vi "observacao_queued.vi"() -> ()   [LabVIEW 2012, in "Shared_160.lvlib"] (continued)
                n273 = local write "sendCommandShutter"(FALSE ("writeShutterLog")) -> ()
                n274 = call "Monta Comando.vi"("Comando"="PARAR", "Dispositivo"="TRAPEIRA" ("Comando"), "Controlador"=w182) -> ()  [unwired: 4 in, 3 out]
              }
            }
            n275 = local read "MOVING"() -> (w97:bool)
            n276 = global write "Global_Telescopio.vi" "Sideral Time"(w114) -> ()
            n277 = Or(x=w96, y=w97) -> (x .or. y?=w95:bool)
            n278 = shared-variable "My Computer\\Shared_160.lvlib\\Beep"(w95) -> ()  [unwired: 1 in, 1 out]
          }
          frame #1 {
            w268 = u16 9 items=["Alarme", "Atencao", "Erro", "Ocupado", "Protecao", "Embreagem", "Tracking", "Var. Track", "Rápido", "Ligeiro", "Médio", "Lento", "Em movimento", ""] ("NomeStatus")
            w269 = u16 9 items=["Alarme", "Atencao", "Erro", "Ocupado", "Protecao", "Embreagem", "Tracking", "Var. Track", "Rápido", "Ligeiro", "Médio", "Lento", "Em movimento", ""] ("NomeStatus")
            w272 = u16 8 items=["Alarme", "Atencao", "Erro", "Ocupado", "Protecao", "Embreagem", "Tracking", "Var. Track", "Rápido", "Ligeiro", "Médio", "Lento", "Em movimento", ""] ("NomeStatus")
            w273 = u16 8 items=["Alarme", "Atencao", "Erro", "Ocupado", "Protecao", "Embreagem", "Tracking", "Var. Track", "Rápido", "Ligeiro", "Médio", "Lento", "Em movimento", ""] ("NomeStatus")
            w279 = 6.283185307179586
            # "Desabilita botões \"Precess\" e \"Clear\"\ndurante o apontamento"
            # "MUDANÇA:\nBit EMBREAGEM trocado pelos bits RAPIDO e LIGEIRO para detectar a retirada do objeto da posição centrada."
            # "MUDANÇA FUTURA:\nTrocar globais de calagem por valores \"latch\" dessas globais. Finalidade: manter display de coordenadas consistentes mesmo quando o usuário zerar as calagens, especialmente a local, para o próximo apontamento."
            # "ATUALIZA INDICADORES DO PAINEL"
            n279 = local read "ChkCalGlobal"() -> (w284:bool)
            n280 = global read "Global_Telescopio.vi" "PosDEC"() -> (w287:dbl)
            n281 = global read "Global_Telescopio.vi" "Sideral Time"() -> (w289:dbl)
            n282 = global read "Global_Telescopio.vi" "ObjCentrado"() -> (w260:bool)
            "ObjCentrado" <- w260
            n283 = global read "Global_Telescopio.vi" "PosAH"() -> (w288:dbl)
            n284 = call "Calcula epoch.vi"() -> ("epoch"=→"Epoch":dbl)  [unwired: 2 in]
            n285 = call "Bit Status AH.vi"("NomeStatus"=w273) -> ("StatBit"=w271:bool)
            n286 = call "Bit Status AH.vi"("NomeStatus"=w268) -> ("StatBit"=w267:bool)
            n287 = call "Bit Status DEC.vi"("NomeStatus"=w272) -> ("StatBit"=w265:bool)
            n288 = call "Bit Status DEC.vi"("NomeStatus"=w269) -> ("StatBit"=w266:bool)
            n289 = Compound Arithmetic op=OR(w271, w267, w265, w266) -> (w270:bool)
            n290 = case shown="True" w270 {
              frame False {
              }
              frame True {
                n291 = global write "Global_Telescopio.vi" "ObjCentrado"(FALSE) -> ()
              }
            }
            n292 = Tick Count (ms)() -> (millisecond timer value=w256:u32)
            n293 = local read "LedPointing"() -> (w255:bool)
            n294 = case shown="True" w260 {
              tunnel: [w366 w383] -> w281
              tunnel: [w365 w382] -> w277
              tunnel: [w368 w386] -> w261
              tunnel: [w367 w384] -> w274
              tunnel: w289 -> [w366 w383]
              tunnel: w288 -> [w371 _]
              tunnel: w287 -> [w370 _]
              tunnel: w284 -> [w369 _]
              tunnel: [w364 w380] -> _
              tunnel: w256 -> [w364 w380]
              frame False {
                n295 = case shown="False" w369 {
                  tunnel: w370 -> [w373 w379]
                  tunnel: [w373 w378] -> w368
                  tunnel: w371 -> [w372 w377]
                  tunnel: [w372 w374] -> w367
                  frame False {
                  }
                  frame True {
                    n296 = global read "Global_Telescopio.vi" "Calagem AH"() -> (w375:dbl)
                    n297 = global read "Global_Telescopio.vi" "Calagem DEC"() -> (w376:dbl)
                    n298 = Subtract(x=w377, y=w375) -> (x-y=w374:dbl)
                    n299 = Subtract(x=w379, y=w376) -> (x-y=w378:dbl)
                  }
                }
                n300 = Subtract(x=w366, y=w367) -> (x-y=w365:dbl)
              }
              frame True {
                # "PROCESSO PRECESSÃO"
                n301 = local read "Temp amb"() -> (w389:string)
                n302 = local read "hum local"() -> (w387:string)
                n303 = local read "MeanDEC"() -> (w390:string)
                n304 = local read "pressão atm"() -> (w388:string)
                n305 = local read "PM_RA"() -> (w385:string)
                n306 = local read "MeanRA"() -> (w391:string)
                n307 = local read "PM_DEC"() -> (w381:string)
                n308 = call "PrecessFortran.vi"("Asc reta"=w391, "Var RA"=w385, "Declinação"=w390, "Temperatura (Kelvin)"=w389, "Pressao atmosferica (mB)"=w388, "Humidade relativa (0 a 1)"=w387, "Var DEC"=w381) -> ("Observed RA (radians)"=w382:dbl, "Observed Dec (radians)"=w386:dbl)  [unwired: 2 in, 5 out]
                n309 = Subtract(x=w383, y=w382) -> (x-y=w384:dbl)
              }
            }
            "AtualDEC" <- w261
            n310 = case shown="True" w260 {
              tunnel: w261 -> [_ w320]
              tunnel: [w317 w319] -> w286
              tunnel: [w317 w318] -> w285
              frame False {
                w317 = 0.0
              }
              frame True {
                n311 = stacked-sequence {
                  seq-local: [w321 _ _] -> [_ _ w359]
                  tunnel: w320 -> [_ w328 _]
                  tunnel: [_ w327 _] -> w319
                  tunnel: [_ w326 _] -> w318
                  frame #0 {
                    n312 = Tick Count (ms)() -> (millisecond timer value=w321:u32)
                  }
                  frame #1 {
                    w329 = u16 3 items=["Alarme", "Atencao", "Erro", "Ocupado", "Protecao", "Embreagem", "Tracking", "Var. Track", "Rápido", "Ligeiro", "Médio", "Lento", "Em movimento", ""] ("NomeStatus")
                    w330 = u16 3 items=["Alarme", "Atencao", "Erro", "Ocupado", "Protecao", "Embreagem", "Tracking", "Var. Track", "Rápido", "Ligeiro", "Médio", "Lento", "Em movimento", ""] ("NomeStatus")
                    # "PROCESSO LEITURA POS_MOTOR"
                    n313 = local read "MOV_IDX_AH"() -> (w324:bool)
                    n314 = local read "MOV_IDX_DEC"() -> (w322:bool)
                    n315 = call "Bit Status AH.vi"("NomeStatus"=w330) -> ("StatBit"=w325:bool)
                    n316 = call "Bit Status DEC.vi"("NomeStatus"=w329) -> ("StatBit"=w323:bool)
                    n317 = case shown="False" w325 {
                      tunnel: w328 -> [w344 _]
                      tunnel: [w343 w358] -> w327
                      tunnel: w324 -> [w342 _]
                      frame False {
                        n318 = case shown="False" w342 {
                          tunnel: w344 -> [w352 _]
                          tunnel: [w348 w357] -> w343
                          frame False {
                            w355 = u16 1 items=["ZERO", "AH", "DEC", "TUBO", "CUP"] ("Controlador")
                            # "RA"
                            # "AH"
                            n319 = call "Get Posic Motor Indexer.vi"("Controlador"=w355) -> ("PosMotor"=w346:dbl)
                            n320 = global read "Global_Telescopio.vi" "AcumPrecRA"() -> (w349:dbl)
                            n321 = Negate(x=w346) -> (-x=w347:dbl)
                            n322 = Subtract(x=w347, y=w349) -> (x-y=w356:dbl)
                            n323 = global read "Global_Telescopio.vi" "AcumAG RA"() -> (w350:dbl)
                            n324 = Cosine(x=w352) -> (cos(x)=w351:dbl)
                            n325 = Absolute Value(x=w351) -> (abs(x)=w345:dbl)
                            n326 = Subtract(x=w356, y=w350) -> (x-y=w354:dbl)
                            n327 = Multiply(x=w345, y=w354) -> (x*y=w353:dbl)
                            n328 = call "Rad to Arcsec.vi"("Radiano"=w353) -> ("Arcsec"=w348:dbl)
                          }
                          frame True {
                            n329 = local read "Offset RA"() -> (w357:dbl)
                          }
                        }
                      }
                      frame True {
                        n330 = local read "Offset RA"() -> (w358:dbl)
                      }
                    }
                    n331 = case shown="False" w323 {
                      tunnel: [w332 w341] -> w326
                      tunnel: w322 -> [w331 _]
                      frame False {
                        n332 = case shown="False" w331 {
                          tunnel: [w333 w340] -> w332
                          frame False {
                            w336 = u16 2 items=["ZERO", "AH", "DEC", "TUBO", "CUP"] ("Controlador")
                            n333 = call "Get Posic Motor Indexer.vi"("Controlador"=w336) -> ("PosMotor"=w338:dbl)
                            n334 = global read "Global_Telescopio.vi" "AcumPrecDEC"() -> (w334:dbl)
                            n335 = Subtract(x=w338, y=w334) -> (x-y=w339:dbl)
                            n336 = global read "Global_Telescopio.vi" "AcumAG DEC"() -> (w335:dbl)
                            n337 = Subtract(x=w339, y=w335) -> (x-y=w337:dbl)
                            n338 = call "Rad to Arcsec.vi"("Radiano"=w337) -> ("Arcsec"=w333:dbl)
                          }
                          frame True {
                            n339 = local read "Offset DEC"() -> (w340:dbl)
                          }
                        }
                      }
                      frame True {
                        n340 = local read "Offset DEC"() -> (w341:dbl)
                      }
                    }
                  }
                  frame #2 {
                    n341 = flat-sequence {
                      tunnel: w359 -> [w360]
                      frame #0 {
                        n342 = Tick Count (ms)() -> (millisecond timer value=w361:u32)
                        n343 = Subtract(x=w361, y=w361) -> (x-y=→"dtAUX2":u32)
                        n344 = Subtract(x=w361, y=w360) -> (x-y=→"dtAUX3":u32)
                      }
                    }
                  }
                }
              }
            }
            "Offset RA" <- w286
            "Offset DEC" <- w285
            n345 = case shown="False" w255 {
              frame False {
                w295 = 0
                n346 = property on="BtPointPrecess" class="Bool"("DisabledEnum"=w295) -> ()  [unwired: 2 in, 2 out]
                n347 = property on="BtPointObjClear" class="Bool"("DisabledEnum"=w295) -> ()  [unwired: 2 in, 2 out]
              }
              frame True {
                w296 = 2
                n348 = property on="BtPointPrecess" class="Bool"("DisabledEnum"=w296) -> ()  [unwired: 2 in, 2 out]
                n349 = property on="BtPointObjClear" class="Bool"("DisabledEnum"=w296) -> ()  [unwired: 2 in, 2 out]
              }
            }
            n350 = call "Normliza_AH.vi"("PosAH"=w274) -> ("Numeric"=w259:dbl)
            n351 = Add(x=w279, y=w277) -> (x+y=w278:dbl)
            n352 = Add(x=w279, y=w281) -> (x+y=w282:dbl)
            n353 = Less Than 0?(x=w281) -> (x < 0?=w283:bool)
            n354 = Less Than 0?(x=w277) -> (x < 0?=w280:bool)
            n355 = Select(t=w282, s=w283, f=w281) -> (s? t:f=w262:dbl)
            n356 = Select(t=w278, s=w280, f=w277) -> (s? t:f=w263:dbl)
            n357 = case shown="True" w260 {
              tunnel: ["" w304] -> w264
              tunnel: w263 -> [_ w301]
              tunnel: w262 -> [_ w302]
              tunnel: w261 -> [_ w303]
              frame False {
              }
              frame True {
                n358 = disable-structure shown="Disabled" {
                  disable-tunnel: w303 -> [w315 _]
                  disable-tunnel: w302 -> [w314 _]
                  disable-tunnel: w301 -> [w313 _]
                  disable-tunnel: [w312 _] -> _
                  frame Disabled {
                    n359 = call "Hora_Limite.vi"("Asc Reta RA rad"=w313, "Sideral Time rad"=w314, "Declinação rad"=w315) -> ("TO Tempo de Observação Horas"=w312:dbl)  [unwired: 2 in]
                  }
                  frame Enabled {
                  }
                }
                n360 = call "Novo_tempo_obs.vi"() -> ("TO rad"=w299:dbl)  [unwired: 10 in, 1 out]
                n361 = Greater Than 0?(x=w299) -> (x > 0?=w298:bool)
                n362 = case shown="True" w298 {
                  tunnel: [w306 w309] -> w300
                  tunnel: w299 -> [w306 w308]
                  frame False {
                  }
                  frame True {
                    n363 = Random Number (0-1)() -> (number: 0 to 1=w310:dbl)
                    n364 = Multiply(x=w310, y=7.27e-05) -> (x*y=w307:dbl)
                    n365 = Add(x=w308, y=w307) -> (x+y=w309:dbl)
                  }
                }
                n366 = call "rad_hms.vi"("TRUE=HORA\nFALSE=GRAU"=TRUE ("TRUE=HORA\nFALSE=GRAU"), "Radiano"=w300) -> ("Hora/Graus Texto Decimal"=w304:string)  [unwired: 3 in]
              }
            }
            "Time to Limit" <- w264
            n367 = call "rad_hms.vi"("TRUE=HORA\nFALSE=GRAU"=TRUE ("TRUE=HORA\nFALSE=GRAU"), "Radiano"=w262) -> ("Hora/Graus Texto Decimal"=w276:string)  [unwired: 3 in]
            "Sideral time" <- w276
            n368 = call "rad_hms.vi"("TRUE=HORA\nFALSE=GRAU"=TRUE, "Radiano"=w263) -> ("Hora/Graus Texto Decimal"=w275:string)  [unwired: 3 in]
            "Right Ascention" <- w275
            n369 = call "rad_hms.vi"("TRUE=HORA\nFALSE=GRAU"=TRUE, "Radiano"=w259) -> ("Hora/Graus Texto Decimal"=w258:string)  [unwired: 3 in]
            "Hour Angle" <- w258
            "Hour Angle 2" <- w258
            n370 = call "rad_hms.vi"("TRUE=HORA\nFALSE=GRAU"=FALSE, "Radiano"=w261) -> ("Hora/Graus Texto Decimal"=w257:string)  [unwired: 3 in]
            "Declination" <- w257
            "DEC" <- w257
            n371 = global write "Global_Telescopio.vi" "Right Ascention"(w275) -> ()
            n372 = global write "Global_Telescopio.vi" "Hour Angle"(w258) -> ()
            n373 = global write "Global_Telescopio.vi" "Sideral time"(w276) -> ()
            n374 = global write "Global_Telescopio.vi" "Declination"(w257) -> ()
            n375 = global write "Global_Telescopio.vi" "AH_now"(w259) -> ()
            n376 = global write "Global_Telescopio.vi" "delta_now"(w261) -> ()
          }
          frame #2 {
            w416 = -0.39330025  # LatOPD rad
            # "ALTERAÇÃO FEITA EM 12/12/2012\nFEITA PARA RESOLVER EXCESSÍVOS\nMOVIMENTOS DO ACOMP.SID. DA\nCÚPULA (DANIEL). A condição de statCUP=0 foi inserida em 08/5/2013-> Só corrige a cúpula se esta estiver parada!"
            # "Horas"
            # "MUDANÇA FUTURA:\nPassar LatOPD para Global"
            # "az"
            # "z"
            # "Cálculo do Azimute da Cúpula e Hab Acompanham. Cúpula"
            # "Lógica de Segurança"
            # "ANGULO ZENITAL"
            n377 = global read "Global_Telescopio.vi" "OffsetCupula"() -> (w425:dbl)
            n378 = global read "Global_Telescopio.vi" "AH_now"() -> (w407:dbl)
            n379 = global read "Global_Telescopio.vi" "delta_now"() -> (w415:dbl)
            n380 = global read "Global_Telescopio.vi" "ErroMaxCup"() -> (w394:i16)
            n381 = global read "Global_Telescopio.vi" "Limite EAST"() -> (w408:dbl)
            n382 = global read "Global_Telescopio.vi" "Limite WEST"() -> (w409:dbl)
            n383 = global read "Global_Telescopio.vi" "PosCUP"() -> (w395:i16)
            "PosCUP" <- w395
            n384 = local read "Tick Cupula"() -> (w399:u32)
            n385 = call "Calculo_do_Azimute_da_Cupula_2.vi"("AH"=w407, "DEC"=w415, "OffsetTCSPD"=w425) -> ("PosCup"=w392:u16)  [unwired: 3 in, 1 out]
            "Azimute cup" <- w392
            n386 = Tick Count (ms)() -> (millisecond timer value=w400:u32)
            n387 = Multiply(x=w407, y=3.8197) -> (x*y=w410:dbl)
            n388 = call "Altura_e_Azimute.vi"("LAT rad"=w416, "DEC rad"=w415, "AH rad"=w407) -> ("AZIMUTE graus"=w413:dbl, "ANG. ZENITAL graus"=w414:dbl, "AZIMUTE rad"=w417:dbl, "ANG. ZENITAL rad"=w418:dbl)  [unwired: 2 out]
            "Azimuth" <- w413
            "Zenital angle" <- w414
            n389 = Greater Or Equal?(x=w400, y=w399) -> (x >= y?=w398:bool)
            n390 = Greater?(x=w410, y=w408) -> (0:w406:bool)
            n391 = Less?(x=w410, y=w409) -> (x < y?=w405:bool)
            n392 = call "Verifica_Correcao_CUP.vi"("Erro max"=w394, "Pos Atual"=w395, "Azimute"=w392) -> ("Corrigir?"=w393:bool)  [unwired: 2 in]
            n393 = Not And(1:w405, 2:w406) -> (0:w402:bool)
            n394 = local read "statCUP"() -> (w397:i32)
            n395 = call "Calcula_Proteção.vi"("Zenital angle rad"=w418, "Azimute rad"=w417) -> ("Z_SEGURANÇA_GRAUS"=w427:dbl, "Prot Segur"=w429:bool, "Z_LIBERA_GRAUS"=w426:dbl, "Z_MAX_GRAUS"=w428:dbl, "Prot Zmax"=w403:bool)
            n396 = Equal To 0?(x=w397) -> (x = 0?=w396:bool)
            n397 = global write "Global_Telescopio.vi" "Z_SEGURANÇA_GRAUS"(w427) -> ()
            n398 = global write "Global_Telescopio.vi" "Zenital angle GRAUS"(w414) -> ()
            n399 = global write "Global_Telescopio.vi" "Azimute GRAUS"(w413) -> ()
            n400 = global write "Global_Telescopio.vi" "Z_MAX_GRAUS"(w428) -> ()
            n401 = global write "Global_Telescopio.vi" "Z_LIBERA_GRAUS"(w426) -> ()
            n402 = Compound Arithmetic op=AND(w393, "DOME", w398, w396) -> (w424:bool)
            n403 = case shown="True" w424 {
              tunnel: w392 -> [_ w438]
              tunnel: FALSE -> [_ w436]
              frame False {
              }
              frame True {
                # "TEMPO CÚPULA"
                # "2m Tempo para novo movimento"
                n404 = local write "Dome on Target"(w436) -> ()
                n405 = Tick Count (ms)() -> (millisecond timer value=w435:u32)
                n406 = To Word Integer(number=w438) -> (16bit integer=w432:i16)
                n407 = local write "statCUP"(1 ("statCUP")) -> ()
                n408 = Add(x=w435, y=u32 120000) -> (x+y=→"Tick Cupula":u32)
                n409 = global write "Global_Telescopio.vi" "TargetCUP"(w432) -> ()
              }
            }
            n410 = Or(x=w402, y=w403) -> (x .or. y?=w404:bool)
            n411 = global read "Global_Telescopio.vi" "LIMITE"() -> (w423:bool)
            n412 = Or(x=w423, y=w404) -> (x .or. y?=w422:bool)
            "Proteção" <- w422
            n413 = call "Borda_Subida_Segurança.vi"("Entrada"=w429) -> ("Boolean"=w430:bool)
            n414 = call "Borda_Subida_Z_max.vi"("Entrada"=w422) -> ("Boolean"=w431:bool)
            n415 = Select(t=u8 2 ("Disabled"), s=w422, f=u8 0 ("Disabled")) -> (s? t:f=w419:u8)
            n416 = property on="MOUNT" class="Bool (strict)"("Disabled"=w419) -> ()  [unwired: 2 in, 2 out]
            n417 = case shown="True" w430 {
              frame False {
              }
              frame True {
                w441 = u16 2 items=["ZERO", "AH", "DEC", "TUBO", "CUP"] ("Controlador")
                w440 = "FREAR" ("Comando")
                w442 = u16 1 items=["ZERO", "AH", "DEC", "TUBO", "CUP"] ("Controlador")
                w439 = "EIXO" ("Dispositivo")
                n418 = call "Monta Comando.vi"("Comando"=w440, "Dispositivo"=w439, "Controlador"=w442) -> ()  [unwired: 4 in, 3 out]
                n419 = call "Monta Comando.vi"("Comando"=w440, "Dispositivo"=w439, "Controlador"=w441) -> ()  [unwired: 4 in, 3 out]
              }
            }
            n420 = case shown="True" w431 {
              frame False {
              }
              frame True {
                w445 = FALSE
                w443 = "Telescópio parado por inclinação excessiva!" ("SYSTEM MESSAGES")
                n421 = local write "LED MOUNT"(w445) -> ()
                n422 = local write "MOUNT"(w445) -> ()
                n423 = global write "Global_Telescopio.vi" "ObjCentrado"(FALSE) -> ()
                n424 = global write "Global_Telescopio.vi" "STOP ALL"(TRUE ("STOP ALL")) -> ()
                n425 = call "Monta_Mensagem.vi"("Mensagem"=w443) -> ()  [unwired: 2 in]
                n426 = call "Salva_systems_messages.vi"("Mensagem"=w443) -> ()  [unwired: 5 in]
              }
            }
            "Led Chave Dome" <- "DOME"
          }
          frame #3 {
            w452 = u32 500 ("millisecond multiple")
            w466 = u16 3 items=["Alarme", "Atencao", "Erro", "Ocupado", "TBD", "LCB", "Trapeira", "Paravento", "DomoRap", "DomoCW", "DomoCCW", "TBD", "Em movimento", "TBD"] ("NomeStatus")
            w480 = u16 3 items=["Alarme", "Atencao", "Erro", "Ocupado", "Protecao", "Embreagem", "Tracking", "Var. Track", "Rápido", "Ligeiro", "Médio", "Lento", "Em movimento", ""] ("NomeStatus")
            w481 = u16 3 items=["Alarme", "Atencao", "Erro", "Ocupado", "Protecao", "Embreagem", "Tracking", "Var. Track", "Rápido", "Ligeiro", "Médio", "Lento", "Em movimento", ""] ("NomeStatus")
            # "04-07-2022\nValor de Erro PROTEC\nalterado de 5 para 10"
            # "MUDANÇA: \nIncluído CASE"
            # "Esse metrônomo determina\no ciclo de 0,5 segundo dos\ncálculos rápidos e totais!"
            # "PROCESSO APONTAMENTO"
            # "MÁQUINA DE ESTADO DO APONTAMENTO"
            # "Seta nome para GO/STOP"
            n427 = global read "Global_Telescopio.vi" "LimiarRapMed"() -> (w482:dbl)
            n428 = global write "Global_Telescopio.vi" "Estado DEC"("statDEC") -> ()
            n429 = global read "Global_Telescopio.vi" "Sideral Time"() -> (w460:dbl)
            n430 = global read "Global_Telescopio.vi" "PosAH"() -> (w485:dbl)
            n431 = global read "Global_Telescopio.vi" "ErroMaxEixo"() -> (w469:dbl)
            n432 = global read "Global_Telescopio.vi" "PosDEC"() -> (w483:dbl)
            n433 = global read "Global_Telescopio.vi" "TargetRA"() -> (w486:dbl)
            n434 = global read "Global_Telescopio.vi" "TargetDEC"() -> (w484:dbl)
            n435 = call "Bit Status DEC.vi"("NomeStatus"=w480) -> ("StatBit"=w468:bool)
            n436 = call "Bit Status AH.vi"("NomeStatus"=w481) -> ("StatBit"=w467:bool)
            n437 = case shown="4" "statDEC" {
              selector: "statDEC" -> [w615 _ _ _ _ _ _ _ _]
              tunnel: [w615 w622 w652 w674 w701 w725 0 ("t") w742 w747] -> w461
              tunnel: w484 -> [_ w621 _ w668 _ _ _ _ _]
              tunnel: w483 -> [_ w617 _ w671 _ _ _ _ _]
              tunnel: w469 -> [_ _ _ w672 _ _ _ _ _]
              tunnel: w482 -> [_ w623 _ _ _ _ _ _ _]
              tunnel: w468 -> [_ w620 _ w667 _ _ _ _ _]
              frame 0, Default {
                w613 = 0 ("CR DEC")
                # "Sem apontamento"
                n438 = call "TickTimeout.vi"() -> ("msTick"=→"TimeoutDEC":u32)  [unwired: 2 in, 2 out]
                n439 = local write "CR DEC"(w613) -> ()
                n440 = local write "C. DEC"(w613) -> ()
              }
              frame 1 {
                # "Envia\nComando"
                n441 = Subtract(x=w621, y=w617) -> (x-y=w619:dbl)
                n442 = Absolute Value(x=w619) -> (abs(x)=w624:dbl)
                n443 = Less?(x=w624, y=w623) -> (x < y?=w618:bool)
                n444 = case shown="False" w618 {
                  tunnel: [w628 3] -> w622
                  tunnel: w621 -> [w627 _]
                  tunnel: w619 -> [w626 _]
                  tunnel: w620 -> [w625 _]
                  frame False {
                    # "destino"
                    # "Fora do"
                    n445 = case shown="False" w625 {
                      tunnel: [w632 w640] -> w628
                      tunnel: w627 -> [w635 _]
                      tunnel: w626 -> [_ _]
                      frame False {
                        w639 = u16 2 items=["ZERO", "AH", "DEC", "TUBO", "CUP"] ("Controlador")
                        # "limpa flag"
                        # "CLP Pronto"
                        n446 = local write "Flag ativo DEC"(FALSE ("Flag ativo DEC")) -> ()
                        n447 = call "rad_hms.vi"("TRUE=HORA\nFALSE=GRAU"=FALSE, "Radiano"=w635) -> ("Hora/Graus Texto Decimal"=w636:string)  [unwired: 3 in]
                        n448 = call "Monta Comando.vi"("Set Point"=w636, "Comando"="MOVER_RAP", "Dispositivo"="EIXO" ("Comando"), "Controlador"=w639) -> ("Erro Comunicação"=w630:bool)  [unwired: 3 in, 2 out]
                        n449 = Select(t=6, s=w630, f=20) -> (s? t:f=w632:i32)
                      }
                      frame True {
                        # "CLP Ocupado"
                        n450 = local read "TimeoutDEC"() -> (w642:u32)
                        n451 = call "TickTimeout.vi"("msInicial"=w642, "msTimeout"=u32 4000) -> ("Timeout"=w641:bool)  [unwired: 2 out]
                        n452 = case shown="False" w641 {
                          tunnel: [1 5] -> w640
                          frame False {
                          }
                          frame True {
                            # "Tratar\nTimeout"
                          }
                        }
                      }
                    }
                  }
                  frame True {
                    # "Dist. pequena p/ mov. rápido"
                    # "Ligar mov. lento"
                    n453 = call "TickTimeout.vi"() -> ("msTick"=w646:u32)  [unwired: 2 in, 2 out]
                    n454 = local write "TimeoutDEC"(w646) -> ()
                  }
                }
                n455 = local write "dec="(FALSE ("dec=")) -> ()
              }
              frame 2 {
                w653 = u16 12 items=["Alarme", "Atencao", "Erro", "Ocupado", "Protecao", "Embreagem", "Tracking", "Var. Track", "Rápido", "Ligeiro", "Médio", "Lento", "Em movimento", ""] ("NomeStatus")
                # "Aguarda fim mov. Rap."
                n456 = call "Bit Status DEC.vi"("NomeStatus"=w653) -> ("StatBit"=w654:bool)
                n457 = case shown="True" w654 {
                  tunnel: [1 w663] -> w651
                  frame False {
                    # "Motor parado.\nTestar se chegou\nao destino"
                    n458 = call "TickTimeout.vi"() -> ("msTick"=w659:u32)  [unwired: 2 in, 2 out]
                    n459 = local write "TimeoutDEC"(w659) -> ()
                  }
                  frame True {
                    # "Ainda movendo...\nAGUARDAR"
                    n460 = local read "Erro PROTEC"() -> (w665:i32)
                    n461 = call "PROTECAO_DEC.vi"() -> ("CONT DEC"=w666:i32)  [unwired: 11 in]
                    "C. DEC" <- w666
                    n462 = Greater Or Equal?(x=w666, y=w665) -> (x >= y?=w661:bool)
                    n463 = Select(t=6, s=w661, f=2) -> (s? t:f=w663:i32)
                  }
                }
                n464 = global read "Global_Telescopio.vi" "Habilita supervisao"() -> (w649:bool)
                n465 = case shown="True" w649 {
                  tunnel: [FALSE w658] -> w648
                  frame False {
                  }
                  frame True {
                    n466 = local read "Erro Lim"() -> (w656:i32)
                    n467 = Greater Or Equal?(x="CR DEC", y=w656) -> (x >= y?=w658:bool)
                  }
                }
                n468 = Select(t=6, s=w648, f=w651) -> (s? t:f=w652:i32)
              }
              frame 3 {
                # "Mov.Lento"
                n469 = Subtract(x=w668, y=w671) -> (x-y=w669:dbl)
                n470 = Absolute Value(x=w669) -> (abs(x)=w673:dbl)
                n471 = Less Or Equal?(x=w673, y=w672) -> (x <= y?=w670:bool)
                n472 = case shown="False" w670 {
                  selector: w670 -> [_ w697]
                  tunnel: [w676 0] -> w674
                  tunnel: w669 -> [w675 _]
                  tunnel: w668 -> [_ w696]
                  tunnel: w667 -> [w677 _]
                  frame False {
                    n473 = case shown="False" w677 {
                      tunnel: [w681 w690] -> w676
                      tunnel: w675 -> [w684 _]
                      frame False {
                        w689 = u16 2 items=["ZERO", "AH", "DEC", "TUBO", "CUP"] ("Controlador")
                        # "limpa flag"
                        # "Mov. lento"
                        n474 = call "TickTimeout.vi"() -> ("msTick"=w683:u32)  [unwired: 2 in, 2 out]
                        n475 = local write "TimeoutDEC"(w683) -> ()
                        n476 = call "rad_hms.vi"("TRUE=HORA\nFALSE=GRAU"=FALSE ("TRUE=HORA\nFALSE=GRAU"), "Radiano"=w684) -> ("Hora/Graus Texto Decimal"=w686:string)  [unwired: 3 in]
                        n477 = local write "Flag ativo DEC"(FALSE ("Flag ativo DEC")) -> ()
                        n478 = call "Monta Comando.vi"("Set Point"=w686, "Comando"="MOVER_REL", "Dispositivo"="EIXO" ("Comando"), "Controlador"=w689) -> ("Erro Comunicação"=w679:bool)  [unwired: 3 in, 2 out]
                        n479 = Select(t=6, s=w679, f=40) -> (s? t:f=w681:i32)
                      }
                      frame True {
                        # "CLP Ocupado"
                        n480 = local read "TimeoutDEC"() -> (w692:u32)
                        n481 = call "TickTimeout.vi"("msInicial"=w692, "msTimeout"=u32 2000) -> ("Timeout"=w691:bool)  [unwired: 2 out]
                        n482 = case shown="False" w691 {
                          tunnel: [3 5] -> w690
                          frame False {
                          }
                          frame True {
                          }
                        }
                      }
                    }
                  }
                  frame True {
                    # "DEC no destino"
                    n483 = local write "LatchDeslocDEC"(w696) -> ()
                    "DEC on Target" <- w697
                  }
                }
              }
              frame 4 {
                w704 = u16 12 items=["Alarme", "Atencao", "Erro", "Ocupado", "Protecao", "Embreagem", "Tracking", "Var. Track", "Rápido", "Ligeiro", "Médio", "Lento", "Em movimento", ""] ("NomeStatus")
                # "Aguarda fim mov. lento"
                n484 = call "Bit Status DEC.vi"("NomeStatus"=w704) -> ("StatBit"=w705:bool)
                n485 = case shown="True" w705 {
                  tunnel: [3 w715] -> w700
                  frame False {
                    # "Motor parado.\nTestar se chegou\nao destino"
                    n486 = call "TickTimeout.vi"() -> ("msTick"=w710:u32)  [unwired: 2 in, 2 out]
                    n487 = local write "TimeoutDEC"(w710) -> ()
                  }
                  frame True {
                    n488 = local read "Erro PROTEC"() -> (w717:i32)
                    n489 = call "PROTECAO_DEC.vi"() -> ("CONT DEC"=w712:i32)  [unwired: 11 in]
                    n490 = local write "C. DEC"(w712) -> ()
                    n491 = Greater Or Equal?(x=w712, y=w717) -> (x >= y?=w714:bool)
                    n492 = local read "TimeoutDEC"() -> (w719:u32)
                    n493 = call "TickTimeout.vi"("msInicial"=w719, "msTimeout"=u32 4000) -> ("Timeout"=w718:bool)  [unwired: 2 out]
                    n494 = case shown="False" w718 {
                      tunnel: [4 5] -> w713
                      frame False {
                      }
                      frame True {
                      }
                    }
                    n495 = Select(t=6, s=w714, f=w713) -> (s? t:f=w715:i32)
                  }
                }
                n496 = global read "Global_Telescopio.vi" "Habilita supervisao"() -> (w702:bool)
                n497 = case shown="True" w702 {
                  tunnel: [FALSE w709] -> w699
                  frame False {
                  }
                  frame True {
                    n498 = local read "CR DEC"() -> (w708:i32)
                    n499 = local read "Erro Lim"() -> (w707:i32)
                    n500 = Greater Or Equal?(x=w708, y=w707) -> (x >= y?=w709:bool)
                  }
                }
                n501 = Select(t=6, s=w699, f=w700) -> (s? t:f=w701:i32)
              }
              frame 5 {
                w730 = u16 2 items=["ZERO", "AH", "DEC", "TUBO", "CUP"] ("Controlador")
                # "Reiniciar apontamento"
                # "Trata Timeout"
                n502 = call "TickTimeout.vi"() -> ("msTick"=w727:u32)  [unwired: 2 in, 2 out]
                n503 = local write "TimeoutDEC"(w727) -> ()
                n504 = call "Monta Comando.vi"("Comando"="PARAR", "Dispositivo"="PROG" ("Comando"), "Controlador"=w730) -> ("Erro Comunicação"=w723:bool)  [unwired: 4 in, 2 out]
                n505 = Select(t=6, s=w723, f=1) -> (s? t:f=w725:i32)
              }
              frame 6 {
                # "PARADA POR ERRO DO CONTROLADOR"
                n506 = stacked-sequence {
                  frame #0 {
                    w733 = u16 2 items=["ZERO", "AH", "DEC", "TUBO", "CUP"] ("Controlador")
                    n507 = call "Monta Comando.vi"("Comando"="PARAR", "Dispositivo"="PROG" ("Comando"), "Controlador"=w733) -> ()  [unwired: 4 in, 3 out]
                    "dec=" <- TRUE ("ah=")
                  }
                  frame #1 {
                    w736 = "Erro de Controlador DEC , REAPONTAR !" ("Mensagem")
                    n508 = local write "Flag de erro p/ apagar lampada"(TRUE ("Flag de erro p/ apagar lampada")) -> ()
                    n509 = call "Monta_Mensagem.vi"("Mensagem"=w736) -> ()  [unwired: 2 in]
                    n510 = call "Salva_systems_messages.vi"("Mensagem"=w736) -> ()  [unwired: 5 in]
                  }
                  frame #2 {
                    w739 = u16 2 items=["ZERO", "AH", "DEC", "TUBO", "CUP"] ("Controlador")
                    # "Em movimento não aceita reset"
                    # "Segundo PARAR por garantia"
                    n511 = call "Monta Comando.vi"("Comando"="PARAR", "Dispositivo"="PROG", "Controlador"=w739) -> ()  [unwired: 4 in, 3 out]
                  }
                }
              }
              frame 20 {
                # "Espera entrar\nem movimento"
                n512 = local read "Flag ativo DEC"() -> (w741:bool)
                n513 = case shown="True" w741 {
                  tunnel: [20 ("t") 2 ("t")] -> w742
                  frame False {
                  }
                  frame True {
                    # "limpa flag"
                    n514 = local write "Flag ativo DEC"(FALSE ("Flag ativo AH")) -> ()
                  }
                }
              }
              frame 40 {
                # "Espera entrar\nem movimento"
                n515 = local read "Flag ativo DEC"() -> (w746:bool)
                n516 = case shown="True" w746 {
                  tunnel: [40 ("t") 4 ("t")] -> w747
                  frame False {
                  }
                  frame True {
                    # "limpa flag"
                    n517 = local write "Flag ativo DEC"(FALSE ("Flag ativo AH")) -> ()
                  }
                }
              }
            }
            n518 = global write "Global_Telescopio.vi" "Estado AH"("statAH") -> ()
            n519 = case shown="1" "statAH" {
              selector: "statAH" -> [w753 _ _ _ _ _ _ _ _ _]
              tunnel: [w753 w762 w790 w806 w830 w858 w883 0 ("t") w899 w904] -> w465
              tunnel: w460 -> [_ w759 _ _ w827 _ _ _ _ _]
              tunnel: w486 -> [_ w758 _ _ w824 _ _ _ _ _]
              tunnel: w485 -> [_ w756 _ _ w826 _ _ _ _ _]
              tunnel: w469 -> [_ _ _ _ w831 _ _ _ _ _]
              tunnel: w482 -> [_ w763 _ _ _ _ _ _ _ _]
              tunnel: w467 -> [_ w760 _ w807 w828 _ _ _ _ _]
              frame 0, Default {
                w751 = 0 ("CR AH")
                # "Sem apontamento"
                n520 = call "TickTimeout.vi"() -> ("msTick"=→"TimeoutAH":u32)  [unwired: 2 in, 2 out]
                n521 = local write "CR AH"(w751) -> ()
                n522 = local write "C. AH"(w751) -> ()
              }
              frame 1 {
                # "Mov.Rapido"
                n523 = call "Calculo_AH.vi"("AH_Telescopio"=w756, "RA_Destino"=w758, "Hora Sideral"=w759) -> ("Dif_Abs_AH"=w757:dbl, "AH_Destino"=w754:dbl)  [unwired: 1 out]
                "AH_Destino" <- w754
                n524 = Less?(x=w757, y=w763) -> (x < y?=w761:bool)
                n525 = case shown="False" w761 {
                  tunnel: w754 -> [w764 _]
                  tunnel: [w765 3] -> w762
                  tunnel: w760 -> [w766 _]
                  frame False {
                    n526 = case shown="True" w766 {
                      tunnel: w764 -> [w772 _]
                      tunnel: [w769 w778] -> w765
                      frame False {
                        w774 = u16 1 items=["ZERO", "AH", "DEC", "TUBO", "CUP"] ("Controlador")
                        # "limpa flag"
                        # "Aguardar\nfim mov."
                        # "Mov. rápido"
                        n527 = local write "Flag ativo AH"(FALSE ("Flag ativo AH")) -> ()
                        n528 = call "rad_hms.vi"("TRUE=HORA\nFALSE=GRAU"=TRUE ("TRUE=HORA\nFALSE=GRAU"), "Radiano"=w772) -> ("Hora/Graus Texto Decimal"=w777:string)  [unwired: 3 in]
                        n529 = call "Monta Comando.vi"("Set Point"=w777, "Comando"="MOVER_RAP", "Dispositivo"="EIXO" ("Comando"), "Controlador"=w774) -> ("Erro Comunicação"=w771:bool)  [unwired: 3 in, 2 out]
                        n530 = Select(t=7, s=w771, f=20) -> (s? t:f=w769:i32)
                      }
                      frame True {
                        # "CLP Ocupado"
                        n531 = local read "TimeoutAH"() -> (w780:u32)
                        n532 = call "TickTimeout.vi"("msInicial"=w780, "msTimeout"=u32 8000) -> ("Timeout"=w779:bool)  [unwired: 2 out]
                        n533 = case shown="True" w779 {
                          tunnel: [1 6] -> w778
                          frame False {
                          }
                          frame True {
                            # "Tratar\nTimeout"
                          }
                        }
                      }
                    }
                  }
                  frame True {
                    # "Ligar acomp. sideral"
                    # "Dist. pequena p/ mov. rápido"
                    n534 = call "TickTimeout.vi"() -> ("msTick"=w784:u32)  [unwired: 2 in, 2 out]
                    n535 = local write "TimeoutAH"(w784) -> ()
                  }
                }
                n536 = local write "ah="(FALSE ("ah=")) -> ()
              }
              frame 2 {
                w792 = u16 12 items=["Alarme", "Atencao", "Erro", "Ocupado", "Protecao", "Embreagem", "Tracking", "Var. Track", "Rápido", "Ligeiro", "Médio", "Lento", "Em movimento", ""] ("NomeStatus")
                # "Aguarda fim mov. Rap."
                n537 = call "Bit Status AH.vi"("NomeStatus"=w792) -> ("StatBit"=w791:bool)
                n538 = case shown="True" w791 {
                  tunnel: [1 w801] -> w789
                  frame False {
                    # "Motor parado.\nTestar se precisa\nde novo cmd. \nde mov. rápido"
                    n539 = call "TickTimeout.vi"() -> ("msTick"=w797:u32)  [unwired: 2 in, 2 out]
                    n540 = local write "TimeoutAH"(w797) -> ()
                  }
                  frame True {
                    # "Aqui também \ncaberia um \nTimeout?"
                    # "Ainda movendo...\nAGUARDAR"
                    n541 = local read "AH_Destino"() -> (w799:dbl)
                    n542 = local read "Erro PROTEC"() -> (w805:i32)
                    n543 = call "PROTECAO_AH.vi"("AH_Destino"=w799) -> ("CONT AH"=w800:i32)  [unwired: 10 in]
                    "C. AH" <- w800
                    n544 = Greater Or Equal?(x=w800, y=w805) -> (x >= y?=w804:bool)
                    n545 = Select(t=7, s=w804, f=2) -> (s? t:f=w801:i32)
                  }
                }
                n546 = global read "Global_Telescopio.vi" "Habilita supervisao"() -> (w787:bool)
                n547 = case shown="True" w787 {
                  tunnel: [FALSE w795] -> w786
                  frame False {
                  }
                  frame True {
                    n548 = local read "Erro Lim"() -> (w794:i32)
                    n549 = Greater Or Equal?(x="CR AH", y=w794) -> (x >= y?=w795:bool)
                  }
                }
                n550 = Select(t=7, s=w786, f=w789) -> (s? t:f=w790:i32)
              }
              frame 3 {
                # "Liga Acomp. Sideral"
                n551 = case shown="True" w807 {
                  tunnel: [w808 w817] -> w806
                  frame False {
                    w812 = TRUE
                    w814 = u16 1 items=["ZERO", "AH", "DEC", "TUBO", "CUP"] ("Controlador")
                    # "Usar mov. lento"
                    # "CLP Pronto - Liga sideral"
                    n552 = call "Monta Comando.vi"("Comando"="LIGAR", "Dispositivo"="SIDERAL" ("Comando"), "Controlador"=w814) -> ("Erro Comunicação"=w810:bool)  [unwired: 4 in, 2 out]
                    n553 = Select(t=7, s=w810, f=4) -> (s? t:f=w808:i32)
                    n554 = call "TickTimeout.vi"() -> ("msTick"=w813:u32)  [unwired: 2 in, 2 out]
                    n555 = local write "LED MOUNT"(w812) -> ()
                    n556 = local write "MOUNT"(w812) -> ()
                    n557 = local write "TimeoutAH"(w813) -> ()
                  }
                  frame True {
                    # "CLP Ocupado"
                    n558 = local read "TimeoutAH"() -> (w819:u32)
                    n559 = call "TickTimeout.vi"("msInicial"=w819, "msTimeout"=u32 8000) -> ("Timeout"=w818:bool)  [unwired: 2 out]
                    n560 = case shown="True" w818 {
                      tunnel: [3 6] -> w817
                      frame False {
                      }
                      frame True {
                        # "Tratar\nTimeout"
                      }
                    }
                  }
                }
              }
              frame 4 {
                # "Mov.Lento"
                n561 = call "Calculo_AH.vi"("AH_Telescopio"=w826, "RA_Destino"=w824, "Hora Sideral"=w827) -> ("Dif_AH"=w823:dbl, "Dif_Abs_AH"=w825:dbl)  [unwired: 1 out]
                n562 = Less?(x=w825, y=w831) -> (x < y?=w829:bool)
                n563 = case shown="False" w829 {
                  selector: w829 -> [_ w854]
                  tunnel: [w833 0] -> w830
                  tunnel: w828 -> [w834 _]
                  tunnel: w824 -> [_ w853]
                  tunnel: w823 -> [w832 _]
                  frame False {
                    n564 = case shown="True" w834 {
                      tunnel: [w837 w847] -> w833
                      tunnel: w832 -> [w841 _]
                      frame False {
                        w843 = u16 1 items=["ZERO", "AH", "DEC", "TUBO", "CUP"] ("Controlador")
                        # "limpa flag"
                        # "Envia Cmd. Mov. Lento"
                        n565 = call "TickTimeout.vi"() -> ("msTick"=w840:u32)  [unwired: 2 in, 2 out]
                        n566 = local write "TimeoutAH"(w840) -> ()
                        n567 = local write "Flag ativo AH"(FALSE ("Flag ativo AH")) -> ()
                        n568 = call "rad_hms.vi"("TRUE=HORA\nFALSE=GRAU"=TRUE ("TRUE=HORA\nFALSE=GRAU"), "Radiano"=w841) -> ("Hora/Graus Texto Decimal"=w846:string)  [unwired: 3 in]
                        n569 = call "Monta Comando.vi"("Set Point"=w846, "Comando"="MOVER_REL", "Dispositivo"="EIXO" ("Comando"), "Controlador"=w843) -> ("Erro Comunicação"=w836:bool)  [unwired: 3 in, 2 out]
                        n570 = Select(t=7, s=w836, f=50) -> (s? t:f=w837:i32)
                      }
                      frame True {
                        # "CLP Ocupado"
                        n571 = local read "TimeoutAH"() -> (w849:u32)
                        n572 = call "TickTimeout.vi"("msInicial"=w849, "msTimeout"=u32 8000) -> ("Timeout"=w848:bool)  [unwired: 2 out]
                        n573 = case shown="False" w848 {
                          tunnel: [4 6] -> w847
                          frame False {
                          }
                          frame True {
                          }
                        }
                      }
                    }
                  }
                  frame True {
                    # "AH on Target"
                    n574 = local write "LatchDeslocRA"(w853) -> ()
                    "RA on Target" <- w854
                  }
                }
              }
              frame 5 {
                w862 = u16 12 items=["Alarme", "Atencao", "Erro", "Ocupado", "Protecao", "Embreagem", "Tracking", "Var. Track", "Rápido", "Ligeiro", "Médio", "Lento", "Em movimento", ""] ("NomeStatus")
                # "Aguarda fim mov. Lento"
                n575 = call "Bit Status AH.vi"("NomeStatus"=w862) -> ("StatBit"=w861:bool)
                n576 = case shown="True" w861 {
                  tunnel: [4 w874] -> w856
                  frame False {
                    # "Motor parado.\nTestar se chegou\nao destino"
                    n577 = call "TickTimeout.vi"() -> ("msTick"=w867:u32)  [unwired: 2 in, 2 out]
                    n578 = local write "TimeoutAH"(w867) -> ()
                  }
                  frame True {
                    # "Trata Timeout"
                    n579 = local read "AH_Destino"() -> (w869:dbl)
                    n580 = local read "Erro PROTEC"() -> (w872:i32)
                    n581 = call "PROTECAO_AH.vi"("AH_Destino"=w869) -> ("CONT AH"=w870:i32)  [unwired: 10 in]
                    n582 = local read "TimeoutAH"() -> (w877:u32)
                    n583 = Greater Or Equal?(x=w870, y=w872) -> (x >= y?=w871:bool)
                    n584 = local write "C. AH"(w870) -> ()
                    n585 = call "TickTimeout.vi"("msInicial"=w877, "msTimeout"=u32 8000) -> ("Timeout"=w876:bool)  [unwired: 2 out]
                    n586 = case shown="False" w876 {
                      tunnel: [5 6] -> w873
                      frame False {
                      }
                      frame True {
                        # "Tratar\nTimeout"
                      }
                    }
                    n587 = Select(t=7, s=w871, f=w873) -> (s? t:f=w874:i32)
                  }
                }
                n588 = global read "Global_Telescopio.vi" "Habilita supervisao"() -> (w860:bool)
                n589 = case shown="True" w860 {
                  tunnel: [FALSE w866] -> w857
                  frame False {
                  }
                  frame True {
                    n590 = local read "Erro Lim"() -> (w864:i32)
                    n591 = local read "CR AH"() -> (w865:i32)
                    n592 = Greater Or Equal?(x=w865, y=w864) -> (x >= y?=w866:bool)
                  }
                }
                n593 = Select(t=7, s=w857, f=w856) -> (s? t:f=w858:i32)
              }
              frame 6 {
                w886 = u16 1 items=["ZERO", "AH", "DEC", "TUBO", "CUP"] ("Controlador")
                # "Reiniciar apontamento"
                # "Trata Timeout"
                n594 = call "TickTimeout.vi"() -> ("msTick"=w885:u32)  [unwired: 2 in, 2 out]
                n595 = call "Monta Comando.vi"("Comando"="PARAR", "Dispositivo"="PROG" ("Comando"), "Controlador"=w886) -> ("Erro Comunicação"=w881:bool)  [unwired: 4 in, 2 out]
                n596 = local write "TimeoutAH"(w885) -> ()
                n597 = Select(t=7, s=w881, f=1) -> (s? t:f=w883:i32)
              }
              frame 7 {
                # "PARADA POR ERRO DO CONTROLADOR"
                n598 = stacked-sequence {
                  frame #0 {
                    w891 = u16 1 items=["ZERO", "AH", "DEC", "TUBO", "CUP"] ("Controlador")
                    n599 = call "Monta Comando.vi"("Comando"="PARAR", "Dispositivo"="PROG" ("Comando"), "Controlador"=w891) -> ()  [unwired: 4 in, 3 out]
                    "ah=" <- TRUE ("ah=")
                  }
                  frame #1 {
                    w894 = "Erro de Controlador RA , REAPONTAR !" ("Mensagem")
                    n600 = call "Monta_Mensagem.vi"("Mensagem"=w894) -> ()  [unwired: 2 in]
                    n601 = call "Salva_systems_messages.vi"("Mensagem"=w894) -> ()  [unwired: 5 in]
                    "Flag de erro p/ apagar lampada" <- TRUE ("Flag de erro p/ apagar lampada")
                  }
                  frame #2 {
                    w898 = u16 1 items=["ZERO", "AH", "DEC", "TUBO", "CUP"] ("Controlador")
                    # "Em movimento não aceita reset"
                    # "Segundo PARAR por garantia"
                    n602 = call "Monta Comando.vi"("Comando"="PARAR", "Dispositivo"="PROG", "Controlador"=w898) -> ()  [unwired: 4 in, 3 out]
                  }
                }
              }
              frame 20 {
                # "Espera entrar\nem movimento"
                n603 = local read "Flag ativo AH"() -> (w900:bool)
                n604 = case shown="True" w900 {
                  tunnel: [20 ("t") 2 ("t")] -> w899
                  frame False {
                  }
                  frame True {
                    # "limpa flag"
                    n605 = local write "Flag ativo AH"(FALSE ("Flag ativo AH")) -> ()
                  }
                }
              }
              frame 50 {
                # "Espera entrar\nem movimento"
                n606 = local read "Flag ativo AH"() -> (w905:bool)
                n607 = case shown="True" w905 {
                  tunnel: [50 ("t") 5 ("t")] -> w904
                  frame False {
                  }
                  frame True {
                    # "limpa flag"
                    n608 = local write "Flag ativo AH"(FALSE ("Flag ativo AH")) -> ()
                  }
                }
              }
            }
            n609 = call "PROTECAO.vi"("Estado In"=w461) -> ("Estado Out"=w447:i32)  [unwired: 2 in]
            n610 = local write "statDEC"(w447) -> ()
            n611 = local read "statCUP"() -> (w471:i32)
            n612 = local read "statDEC"() -> (w472:i32)
            n613 = local read "statAH"() -> (w473:i32)
            n614 = call "PROTECAO.vi"("Estado In"=w465) -> ("Estado Out"=w464:i32)  [unwired: 2 in]
            n615 = global read "Global_Telescopio.vi" "Botão GO = STOP"() -> (w459:bool)
            n616 = local write "statAH"(w464) -> ()
            n617 = Compound Arithmetic op=ADD(w471, w473, w472) -> (w475:i32)
            n618 = call "Bit Status CUP.vi"("NomeStatus"=w466) -> ("StatBit"=w479:bool)
            n619 = global read "Global_Telescopio.vi" "PosCUP"() -> (w478:i16)
            n620 = global read "Global_Telescopio.vi" "ErroMaxCup"() -> (w476:i16)
            n621 = global read "Global_Telescopio.vi" "TargetCUP"() -> (w477:i16)
            n622 = global write "Global_Telescopio.vi" "Estado CUP"("statCUP") -> ()
            n623 = Equal To 0?(x=w475) -> (x = 0?=w474:bool)
            n624 = And(x=w474, y=w459) -> (x .and. y?=w470:bool)
            n625 = case shown="7" "statCUP" {
              selector: "statCUP" -> [w498 _ _ _ _ _ _ _]
              tunnel: [w498 w502 w549 1 w559 w580 w590 w608] -> w463
              tunnel: w479 -> [_ w504 _ _ w561 _ w586 _]
              tunnel: w478 -> [_ w508 _ _ _ _ _ _]
              tunnel: w477 -> [_ w503 _ _ _ _ _ _]
              tunnel: w476 -> [_ w506 _ _ _ _ _ _]
              frame 0, Default {
                # "Sem movimento"
                n626 = call "TickTimeout.vi"() -> ("msTick"=→"TimeoutCUP":u32)  [unwired: 2 in, 2 out]
              }
              frame 1 {
                # "Envia\nComando"
                n627 = local read "LedPointing"() -> (w499:bool)
                n628 = local read "DOME"() -> (w500:bool)
                n629 = Subtract(x=w503, y=w508) -> (x-y=w507:i16)
                n630 = Absolute Value(x=w507) -> (abs(x)=w509:i16)
                n631 = Less Or Equal?(x=w509, y=w506) -> (x <= y?=w505:bool)
                n632 = case shown="True" w505 {
                  tunnel: w504 -> [w515 w539]
                  tunnel: w503 -> [w514 _]
                  tunnel: [w513 w540] -> w502
                  tunnel: "ChkDomeEnable" -> [w510 w538]
                  tunnel: w500 -> [w512 w537]
                  tunnel: w499 -> [w511 w536]
                  frame False {
                    # "CUP fora pos."
                    n633 = case shown="False" w515 {
                      tunnel: w514 -> [w522 _]
                      tunnel: [w520 w530] -> w513
                      tunnel: w512 -> [w519 _]
                      tunnel: w511 -> [w517 _]
                      tunnel: w510 -> [w516 _]
                      frame False {
                        # "CLP Pronto"
                        n634 = Number To Decimal String(number=w522) -> (decimal integer string=w521:string)  [unwired: 1 in]
                        n635 = Select(t=w516, s=w517, f=w519) -> (s? t:f=w518:bool)
                        n636 = case shown="False" w518 {
                          tunnel: [0 2] -> w520
                          tunnel: w521 -> [_ w525]
                          frame False {
                            # "Cúpula Desabilitada"
                            # "Também não verifica\nTrapeira e Paravento"
                          }
                          frame True {
                            w527 = u16 4 items=["ZERO", "AH", "DEC", "TUBO", "CUP"] ("Controlador")
                            n637 = call "TickTimeout.vi"() -> ("msTick"=w524:u32)  [unwired: 2 in, 2 out]
                            n638 = local write "TimeoutCUP"(w524) -> ()
                            n639 = global write "Global_Telescopio.vi" "T cup"(w524) -> ()
                            n640 = call "Monta Comando.vi"("Set Point"=w525, "Comando"="MOVER", "Dispositivo"="DOMO" ("Comando"), "Controlador"=w527) -> ()  [unwired: 3 in, 3 out]
                          }
                        }
                      }
                      frame True {
                        # "CLP Busy"
                        n641 = local read "TimeoutCUP"() -> (w532:u32)
                        n642 = call "TickTimeout.vi"("msInicial"=w532, "msTimeout"=u32 5000) -> ("Timeout"=w531:bool)  [unwired: 2 out]
                        n643 = case shown="True" w531 {
                          tunnel: [1 3] -> w530
                          frame False {
                          }
                          frame True {
                          }
                        }
                      }
                    }
                  }
                  frame True {
                    # "CUP no destino"
                    n644 = case shown="True" w536 {
                      tunnel: [0 w544] -> w540
                      tunnel: w539 -> [_ _]
                      tunnel: w538 -> [_ w543]
                      tunnel: w537 -> [w541 _]
                      frame False {
                        # "Não está apontando (chave Dome Enable foi ativada)"
                        # "Não verifica\nTrapeira e\nParavento"
                        n645 = local write "Dome on Target"(w541) -> ()
                      }
                      frame True {
                        # "Está apontando"
                        n646 = case shown="True" w543 {
                          tunnel: [0 4] -> w544
                          frame False {
                            # "Não verifica\nTrapeira e\nParavento"
                          }
                          frame True {
                            # "Verifica Trapeira e\nParavento"
                            n647 = call "TickTimeout.vi"() -> ("msTick"=w546:u32)  [unwired: 2 in, 2 out]
                            n648 = local write "TimeoutCUP"(w546) -> ()
                            n649 = global write "Global_Telescopio.vi" "T cup"(w546) -> ()
                          }
                        }
                      }
                    }
                  }
                }
              }
              frame 2 {
                w548 = u16 12 items=["Alarme", "Atencao", "Erro", "Ocupado", "TBD", "LCB", "Trapeira", "Paravento", "DomoRap", "DomoCW", "DomoCCW", "TBD", "Em movimento", "TBD"] ("NomeStatus")
                # "Aqui também caberia um Timeout?"
                # "Aguarda parada motor"
                n650 = call "Bit Status CUP.vi"("NomeStatus"=w548) -> ("StatBit"=w550:bool)
                n651 = case shown="True" w550 {
                  tunnel: [1 2] -> w549
                  frame False {
                    # "Motor parado.\nTestar se chegou\nao destino"
                    n652 = call "TickTimeout.vi"() -> ("msTick"=w551:u32)  [unwired: 2 in, 2 out]
                    n653 = local write "TimeoutCUP"(w551) -> ()
                    n654 = global write "Global_Telescopio.vi" "T cup"(w551) -> ()
                  }
                  frame True {
                    # "Ainda movendo...\nAGUARDAR"
                  }
                }
              }
              frame 3 {
                w557 = u16 4 items=["ZERO", "AH", "DEC", "TUBO", "CUP"] ("Controlador")
                # "Trata Timeout"
                n655 = call "TickTimeout.vi"() -> ("msTick"=w554:u32)  [unwired: 2 in, 2 out]
                n656 = local write "TimeoutCUP"(w554) -> ()
                n657 = global write "Global_Telescopio.vi" "T cup"(w554) -> ()
                n658 = call "Monta Comando.vi"("Comando"="PARAR", "Dispositivo"="PROG" ("Comando"), "Controlador"=w557) -> ()  [unwired: 4 in, 3 out]
              }
              frame 4 {
                w560 = u16 7 items=["Alarme", "Atencao", "Erro", "Ocupado", "TBD", "LCB", "Trapeira", "Paravento", "DomoRap", "DomoCW", "DomoCCW", "TBD", "Em movimento", "TBD"] ("NomeStatus")
                # "Verifica Paravento"
                n659 = call "Bit Status CUP.vi"("NomeStatus"=w560) -> ("StatBit"=w564:bool)
                n660 = Not(x=w564) -> (.not. x?=w565:bool)
                n661 = And(x=w565, y="ChkWindDown") -> (x .and. y?=w562:bool)
                n662 = case shown="True" w562 {
                  tunnel: w561 -> [_ w568]
                  tunnel: [6 w567] -> w559
                  frame False {
                    # "Paravento abaixado\nou desabilitado"
                  }
                  frame True {
                    # "Descer Parav."
                    n663 = case shown="True" w568 {
                      tunnel: [5 w573] -> w567
                      frame False {
                        w572 = u16 4 items=["ZERO", "AH", "DEC", "TUBO", "CUP"] ("Controlador")
                        # "Aguardar abaixa/o Parav."
                        # "CLP Pronto"
                        n664 = call "Monta Comando.vi"("Comando"="DESCER", "Dispositivo"="PARAVENTO" ("Comando"), "Controlador"=w572) -> ()  [unwired: 4 in, 3 out]
                      }
                      frame True {
                        # "CLP Busy"
                        n665 = local read "TimeoutCUP"() -> (w575:u32)
                        n666 = call "TickTimeout.vi"("msInicial"=w575, "msTimeout"=u32 5000) -> ("Timeout"=w574:bool)  [unwired: 2 out]
                        n667 = case shown="True" w574 {
                          tunnel: [4 3] -> w573
                          frame False {
                          }
                          frame True {
                          }
                        }
                      }
                    }
                  }
                }
              }
              frame 5 {
